vi "Compute Optimal Nanotime Bin Sizes.vi"(9 "Max # Gates":i32, 11 "PicoQuant Data File Information":T1) -> (0 "Residual Bin Fraction":dbl, 1 "Gate Step/Width (res unit)":dbl, 2 "Gate Step & Width (s)":dbl, 3 "Optimal # Gates":i32, 4 "Mp":dbl)   [LabVIEW 2021, in "PTU Files.lvlib"]
uses:
  PTU Files.lvlib
  <userlib>/_OpenG.lib/array/array.llb/openg_array.lvlib
  <userlib>/_OpenG.lib/array/array.llb/Remove Duplicates from 1D Array (DBL)__ogtk.vi
  <userlib>/_OpenG.lib/array/array.llb/Index 1D Array Elements (I32)__ogtk.vi
  <userlib>/_OpenG.lib/array/array.llb/Search 1D Array (DBL)__ogtk.vi
  <userlib>/_OpenG.lib/array/array.llb/Sort 1D Array (DBL)__ogtk.vi
  PicoQuant File Information.ctl
  PicoQuant Software Information.ctl
  PicoQuant Remote Request Information.ctl
  PicoQuant Input Channels.ctl
  PicoQuant Markers.ctl
  PicoQuant Modules.ctl
  PicoQuant Router Channels.ctl
  PicoQuant Hardware Information.ctl
  PicoQuant Measurement Information.ctl
  PicoQuant Image Information.ctl
  PicoQuant Results Format.ctl
  PicoQuant Measurement Results.ctl
  PicoQuant Data File Information.ctl
panel:
  out "Number of Bins":i32[](array[numeric])
  out "Number of leftover dt":dbl[](array[numeric])
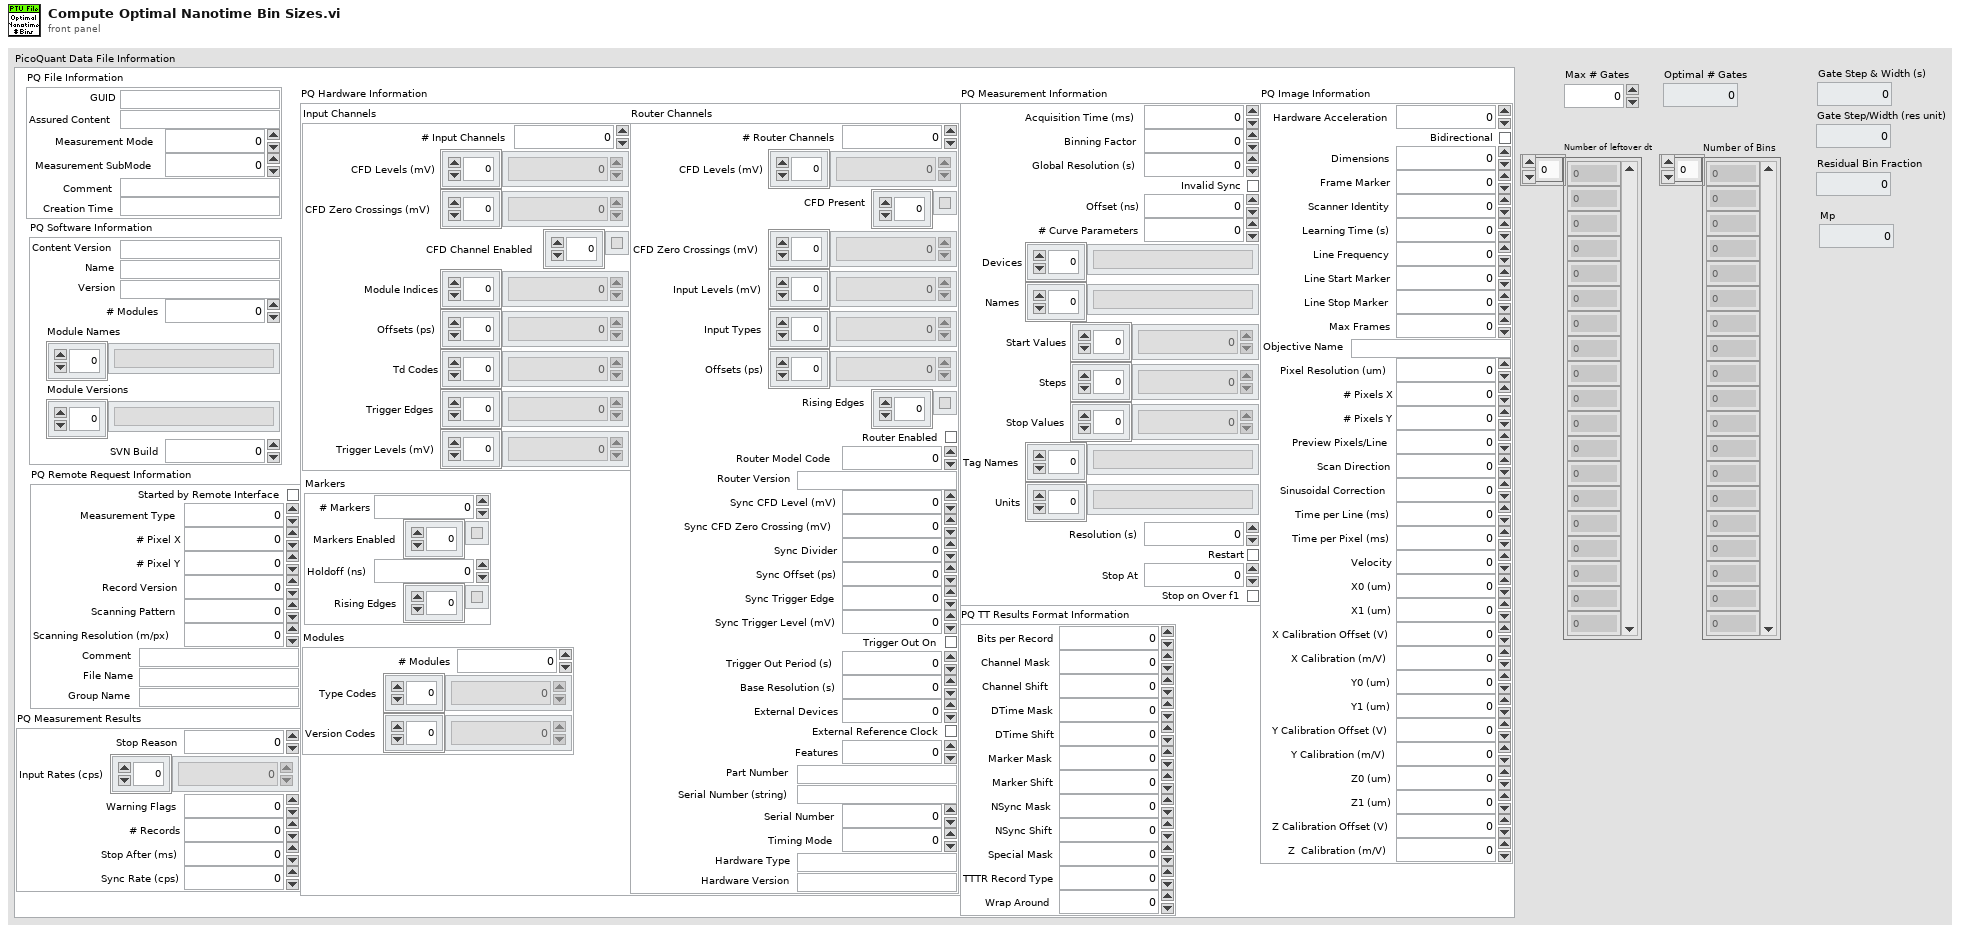
[diagram p1: front panel]
types:
  T1 = typedef "PTU Files.lvlib/PicoQuant Data File Information.ctl" = cluster{"PQ File Information":T2, "PQ Software Information":T3, "PQ Remote Request Information":T4, "PQ Hardware Information":T5, "PQ Measurement Information":T10, "PQ Image Information":T11, "PQ TT Results Format Information":T12, "PQ Measurement Results":T13}
  T2 = typedef "PTU Files.lvlib/PicoQuant File Information.ctl" = cluster{"GUID":string, "Assured Content":string, "Measurement Mode":i64, "Measurement SubMode":i64, "Comment":string, "Creation Time":string}
  T3 = typedef "PTU Files.lvlib/PicoQuant Software Information.ctl" = cluster{"Content Version":string, "Name":string, "Version":string, "# Modules":i64, "Module Names":string[], "Module Versions":string[], "SVN Build":i64}
  T4 = typedef "PTU Files.lvlib/PicoQuant Remote Request Information.ctl" = cluster{"Started by Remote Interface":bool, "Measurement Type":i64, "# Pixel X":i64, "# Pixel Y":i64, "Record Version":i64, "Scanning Pattern":i64, "Scanning Resolution (m/px)":dbl, "Comment":string, "File Name":string, "Group Name":string}
  T5 = typedef "PTU Files.lvlib/PicoQuant Hardware Information.ctl" = cluster{"Input Channels":T6, "Markers":T7, "Modules":T8, "Router Channels":T9}
  T6 = typedef "PTU Files.lvlib/PicoQuant Input Channels.ctl" = cluster{"# Input Channels":i64, "CFD Levels (mV)":i64[], "CFD Zero Crossings (mV)":i64[], "CFD Channel Enabled":bool[], "Module Indices":i64[], "Offsets (ps)":i64[], "Td Codes":i64[], "Trigger Edges":i64[], "Trigger Levels (mV)":i64[]}
  T7 = typedef "PTU Files.lvlib/PicoQuant Markers.ctl" = cluster{"# Markers":i64, "Markers Enabled":bool[], "Holdoff (ns)":i64, "Rising Edges":bool[]}
  T8 = typedef "PTU Files.lvlib/PicoQuant Modules.ctl" = cluster{"# Modules":i64, "Type Codes":i64[], "Version Codes":i64[]}
  T9 = typedef "PTU Files.lvlib/PicoQuant Router Channels.ctl" = cluster{"# Router Channels":i64, "CFD Levels (mV)":i64[], "CFD Present":bool[], "CFD Zero Crossings (mV)":i64[], "Input Levels (mV)":i64[], "Input Types":i64[], "Offsets (ps)":i64[], "Rising Edges":bool[], "Router Enabled":bool, "Router Model Code":i64, "Router Version":string, "Sync CFD Level (mV)":i64, "Sync CFD Zero Crossing (mV)":i64, "Sync Divider":i64, "Sync Offset (ps)":i64, "Sync Trigger Edge":i64, "Sync Trigger Level (mV)":i64, "Trigger Out On":bool, "Trigger Out Period (s)":dbl, "Base Resolution (s)":dbl, "External Devices":i64, "External Reference Clock":bool, "Features":u64, "Part Number":string, "Serial Number (string)":string, "Serial Number":i64, "Timing Mode":i64, "Hardware Type":string, "Hardware Version":string}
  T10 = typedef "PTU Files.lvlib/PicoQuant Measurement Information.ctl" = cluster{"Acquisition Time (ms)":i64, "Binning Factor":i64, "Global Resolution (s)":dbl, "Invalid Sync":bool, "Offset (ns)":u64, "# Curve Parameters":u64, "Devices":string[], "Names":string[], "Start Values":dbl[], "Steps":dbl[], "Stop Values":dbl[], "Tag Names":string[], "Units":string[], "Resolution (s)":dbl, "Restart":bool, "Stop At":u64, "Stop on Over f1":bool}
  T11 = typedef "PTU Files.lvlib/PicoQuant Image Information.ctl" = cluster{"Hardware Acceleration":i64, "Bidirectional":bool, "Dimensions":i64, "Frame Marker":i64, "Scanner Identity":i64, "Learning Time (s)":i64, "Line Frequency":dbl, "Line Start Marker":i64, "Line Stop Marker":i64, "Max Frames":i64, "Objective Name":string, "Pixel Resolution (um)":dbl, "# Pixels X":i64, "# Pixels Y":i64, "Preview Pixels/Line":i64, "Scan Direction":i64, "Sinusoidal Correction":i64, "Time per Line (ms)":dbl, "Time per Pixel (ms)":i64, "Velocity":i64, "X0 (um)":dbl, "X1 (um)":dbl, "X Calibration Offset (V)":dbl, "X Calibration (m/V)":dbl, "Y0 (um)":dbl, "Y1 (um)":dbl, "Y Calibration Offset (V)":dbl, "Y Calibration (m/V)":dbl, "Z0 (um)":dbl, "Z1 (um)":dbl, "Z Calibration Offset (V)":dbl, "Z  Calibration (m/V)":dbl}
  T12 = typedef "PTU Files.lvlib/PicoQuant Results Format.ctl" = cluster{"Bits per Record":i64, "Channel Mask":i64, "Channel Shift ":i64, "DTime Mask":i64, "DTime Shift":i64, "Marker Mask":i64, "Marker Shift":i64, "NSync Mask":i64, "NSync Shift":i64, "Special Mask":i64, "TTTR Record Type":i64, "Wrap Around":i64}
  T13 = typedef "PTU Files.lvlib/PicoQuant Measurement Results.ctl" = cluster{"Stop Reason":i64, "Input Rates (cps)":i64[], "Warning Flags":u64, "# Records":i64, "Stop After (ms)":i64, "Sync Rate (cps)":i64}
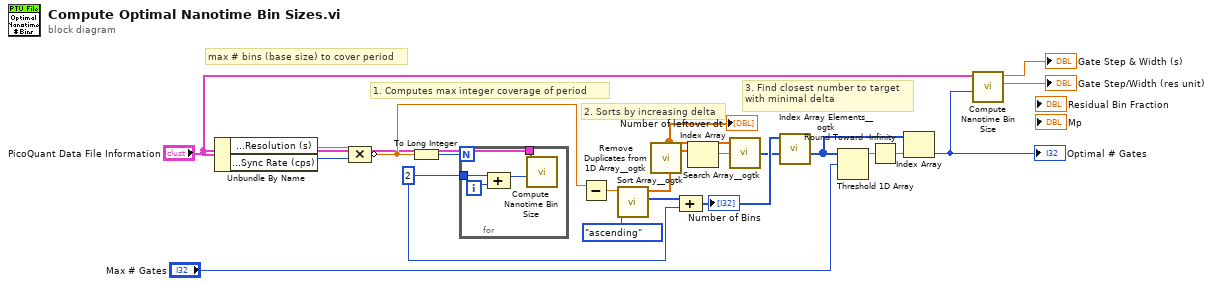
[diagram p0: block diagram]
diagram:
  w15 = 2 ("value")
  # "3. Find closest number to target\nwith minimal delta"
  # "2. Sorts by increasing delta"
  # "1. Computes max integer coverage of period"
  # "max # bins (base size) to cover period"
  n1 = Unbundle By Name("PicoQuant Data File Information") -> ("PQ Measurement Information.Resolution (s)"=w20:dbl, "PQ Measurement Results.Sync Rate (cps)"=w21:i64)
  n2 = Compound Arithmetic op=MULTIPLY(w20, w21) -> (invert w14:dbl)
  n3 = To Long Integer(number=w14) -> (32bit integer=w19:i32)
  n4 = for {
    N: w19 -> [_]
    tunnel: w15 -> [w25]
    tunnel: "PicoQuant Data File Information" -> [w23]
    i -> [w24]
    n5 = Compound Arithmetic op=ADD(w25, w24) -> (w22:i32)
    n6 = call "Compute Nanotime Bin Size.vi"("# Gates"=w22, "PicoQuant Data File Information"=w23) -> ()  [unwired: 7 in, 3 out]
  }
  n7 = Subtract(x=w14) -> (x-y=w18:dbl)  [unwired: 1 in]
  n8 = call-poly <userlib>:"Sort Array__ogtk.vi"("Order"=enum16{"ascending", "descending"}."ascending", "Array in"=w18) -> ("Sorted Pointers"=w16:i32[], "Sorted Array out"=w12:dbl[])  [unwired: 8 in]
  "Number of leftover dt" <- w12
  n9 = call-poly <userlib>:"Remove Duplicates from 1D Array__ogtk.vi"("Input Array"=w12) -> ("Output Array"=w13:dbl[])  [unwired: 1 out]
  n10 = Compound Arithmetic op=ADD(w16, w15) -> (w10:i32[])
  "Number of Bins" <- w10
  n11 = Index Array(array=w13) -> (element=w11:dbl)  [unwired: 1 in]
  n12 = call-poly <userlib>:"Search Array__ogtk.vi"("Array"=w12, "Element Data"=w11) -> ("Indices of Elements"=w9:i32[])  [unwired: 7 in]
  n13 = call-poly <userlib>:"Index Array Elements__ogtk.vi"("indices"=w9, "array"=w10) -> ("elements"=w7:i32[])  [unwired: 9 in]
  n14 = Threshold 1D Array(2:"Max # Gates", 3:w7) -> (0:w6:dbl)  [unwired: 1 in]
  n15 = Round Toward -Infinity(1:w6) -> (0:w1:dbl)
  n16 = Index Array(array=w7, index=w1) -> (element=w5:i32)
  "Optimal # Gates" <- w5
  n17 = call "Compute Nanotime Bin Size.vi"("# Gates"=w5, "PicoQuant Data File Information"="PicoQuant Data File Information") -> ("p (# native bins per user bin)"=→"Gate Step/Width (res unit)":dbl, "user bin size (Gate Step & Width) (s)"=→"Gate Step & Width (s)":dbl)  [unwired: 7 in, 1 out]
